vi "TestNetOConvert.vi"() -> ()   [LabVIEW 2017]
uses:
  C:/Code/CMCryoSysCode/Expose/COM/CSCom/CSCom/bin/Release/CSCom.dll
  COM/CSCom/CSCom/bin/Release/CSCom.dll
panel:
  out "Get direct":dbl
  out "Convert via labview":dbl
  out "Create":dbl
  in  "cnt":i32
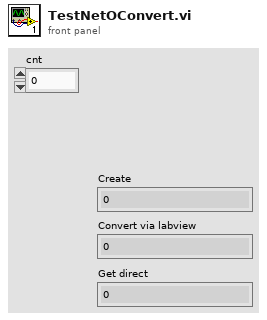
[diagram p1: front panel]
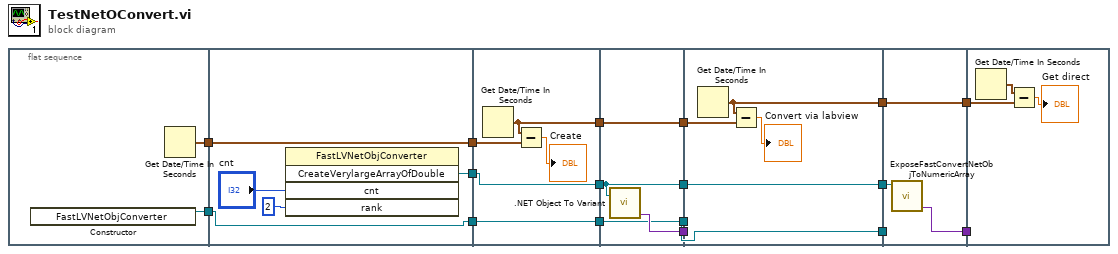
[diagram p0: block diagram]
diagram:
  n1 = flat-sequence {
    tunnel: [w19] -> w16
    tunnel: [w18] -> w2
    tunnel: [w24] -> w17
    tunnel: w16 -> [w24]
    tunnel: [w23] -> w3
    tunnel: w2 -> [w23]
    tunnel: [w20] -> w1
    tunnel: w17 -> [w29]
    tunnel: [w27] -> w15
    tunnel: [w25] -> w10
    tunnel: [w26] -> w4
    tunnel: w3 -> [w26]
    tunnel: w1 -> [w25]
    tunnel: w15 -> [w33]
    tunnel: [w33] -> w14
    tunnel: [w32] -> w11
    tunnel: w10 -> [w31]
    tunnel: [w31] -> w9
    tunnel: [w30] -> w5
    tunnel: w4 -> [w30]
    tunnel: w14 -> [w37]
    tunnel: [w36] -> w13
    tunnel: w11 -> [_]
    tunnel: w9 -> [w35]
    tunnel: [w35] -> w8
    tunnel: [w34] -> w6
    tunnel: w5 -> [w34]
    tunnel: w13 -> [w41]
    tunnel: [w41] -> w12
    tunnel: w8 -> [w40]
    tunnel: [w39] -> w7
    tunnel: w6 -> [_]
    tunnel: w12 -> [w42]
    tunnel: w7 -> [_]
    frame #0 {
      n2 = constructor class="FastLVNetObjConverter"() -> (reference out=w18:refnum<k24>)  [unwired: 3 in, 2 out]
      n3 = Get Date/Time In Seconds() -> (seconds since 1Jan1904=w19:timestamp)
    }
    frame #1 {
      n4 = invoke class="FastLVNetObjConverter" method="CreateVerylargeArrayOfDouble"("cnt"="cnt", "rank"=2) -> ("CreateVerylargeArrayOfDouble"=w20:refnum<k24>)  [unwired: 3 in, 4 out]
    }
    frame #2 {
      n5 = Get Date/Time In Seconds() -> (seconds since 1Jan1904=w27:timestamp)
      n6 = Subtract(x=w27, y=w29) -> (x-y=→"Create":dbl)
    }
    frame #3 {
      n7 = call <vilib>:".NET Object To Variant.vi"(".NET object"=w31) -> ("variant"=w32:variant)  [unwired: 1 in, 1 out]
    }
    frame #4 {
      n8 = Get Date/Time In Seconds() -> (seconds since 1Jan1904=w36:timestamp)
      n9 = Subtract(x=w36, y=w37) -> (x-y=→"Convert via labview":dbl)
    }
    frame #5 {
      n10 = call "ExposeFastConvertNetObjToNumericArray.vi"(".NET Refnum in"=w40) -> ("Array"=w39:variant)  [unwired: 10 in]
    }
    frame #6 {
      n11 = Get Date/Time In Seconds() -> (seconds since 1Jan1904=w43:timestamp)
      n12 = Subtract(x=w43, y=w42) -> (x-y=→"Get direct":dbl)
    }
  }
